vi "Intake Loop.vi"   [LabVIEW 2015]
uses:
  Common Code/Intake States.ctl
  Robot Global Data.vi
types:
  T1 = typedef "Dashboard Control Data.ctl" = cluster{"Shooter Presets":T2, "Encoder Control":T4, "Steer PID output":cluster{"output high":dbl, "output low":dbl}, " Steer PID gains":cluster{"proportional gain (Kc)":dbl, "integral time (Ti, min)":dbl, "derivative time (Td, min)":dbl}, "Drivetrain Settings":T5, "Vision Packet":T6, "Dashboard Drivetrain Command":T7, "Info/Command Cluster":T9, "Ball Vision Packet":T10, "Intake Presets":T12, "Intake Encoder Control":T14, "Climb Presets":T15, "Goal Output Range":cluster{"output high":dbl, "output low":dbl}, "Enabled Systems":T16, "Auton Presets":T17, "Pressure M":dbl, "Pressure B":dbl, "Vision Timeout":dbl}
  T2 = typedef "Shooter Presets.ctl" = cluster{"Batter Shot":T3, "Deep Middle":T3, "Manual Shot":T3, "Left Ticks Per Rotation":dbl, "Right Ticks Per Rotation":dbl, "Low Bar Shot":T3, "Shooter RPM Tolerance":dbl, "Trigger Power":dbl, "Fire from Load Delay":i32, "Max Angle":dbl, "Min Angle":dbl, "Angle PID gains":cluster{"P":dbl, "I":dbl, "D":dbl}, "Angle Output":cluster{"output high":dbl, "output low":dbl}, "Shooter Angle Tolerance":dbl, "Vision Shoot x^2":dbl, "Vision Shoot x":dbl, "Feed Forward Max Accel":dbl, "Feed Forward Kv":dbl, "Backwards Trigger":dbl, "Shot Finish Delay (ms)":dbl, "Angle Max Current":dbl, "Angle Current Trip Time":dbl, "Intake Angle":dbl, "Vision Shoot c":dbl, "Reset?":bool, "Button Release Delay":dbl, "Angle Pot x":dbl, "Angle Pot c":dbl, "Ignore Angle?":bool, "Max RPM":dbl, "Safty Frist Angle":dbl, "Intake Danger Height":dbl, "Angle Pot B":i32, "Angle Pot M":dbl, "FF Finish RPM":dbl, "RPM PID Right":cluster{"P":dbl, "I":dbl, "D":dbl, "FF":dbl}, "RPM PID Left":cluster{"P":dbl, "I":dbl, "D":dbl, "FF":dbl}, "Backwards RPM":dbl, "Vision RPM":dbl, "Run Wheels Backward Delay":u32, "Cleat Shot":T3}
  T3 = typedef "Shot Presets.ctl" = cluster{"L":dbl, "R":dbl, "A":dbl}
  T4 = typedef "Encoder Control.ctl" = cluster{"Right Tick Constant":dbl, "Left Tick Constant":dbl, "Reset?":bool, "Y Dist":cluster{"PID gains":cluster{"proportional gain (Kc)":dbl, "integral time (Ti, min)":dbl, "derivative time (Td, min)":dbl}}, "Y Stop Thresh":dbl, "Y Stop Speed":dbl}
  T5 = typedef "Drivetrain Settings.ctl" = cluster{"Gyro Tolerance":dbl, "Throttle Ramp (ms)":dbl, "Kv":dbl, "Ka":dbl, "Feed Forward P":dbl, "Feed Forward D":dbl, "Goal Vision PID gains":cluster{"proportional gain (Kc)":dbl, "integral time (Ti, min)":dbl, "derivative time (Td, min)":dbl}, "Goal Detection Window":dbl, "Creep Rate":dbl, "Vision Throttle Threshold":dbl, "Min Turn Output":dbl, "Left Batter Angle":dbl, "Right Batter Angle":dbl}
  T6 = typedef "Goal Vision Packet.ctl" = cluster{"Distance":dbl, "Center X":dbl, "Center Y":dbl, "Found Target?":bool, "Robot Center":dbl, "Angle":dbl}
  T7 = typedef "Dashboard Drivetrain Command.ctl" = cluster{"Drivetrain Vision":T8}
  T8 = typedef "Drivetrain Vision.ctl" = cluster{"Goal Window":dbl, "Ball Window":dbl}
  T9 = typedef "Ball Tracking Command Cluster.ctl" = cluster{"Distance to Ball":dbl, "Desired Angle":dbl, "Command":enum16{"Turn to Ball", "Turn to Angle", "Get Distance"}, "Pixels from Center":dbl}
  T10 = typedef "Ball Vision Packet.ctl" = cluster{"Ball Detected?":bool, "Distance to Ball":dbl, "Desired Angle":dbl, "Pixels from Center":dbl, "Tracking mode":T11}
  T11 = typedef "Tracking Mode.ctl" = enum16{"Turn to Ball", "Turn to Angle"}
  T12 = typedef "Intake Presets.ctl" = cluster{"Intake Speed":dbl, "Outake Speed":dbl, "Low Height":dbl, "Half Height":dbl, "Full Height":dbl, "Angle Speed":dbl, "Angle Tolerance":dbl, "Encoder Scale":dbl, "Load Height":dbl, "Output Range":T13, "Rotation Power Max/Min":dbl, "MaxCurrent":dbl, "Intake Trip Time":dbl, "Idle Height":dbl, "Max Height":dbl, "Reset Encoders?":bool, "PID gains":cluster{"proportional gain (Kc)":dbl, "integral time (Ti, min)":dbl, "derivative time (Td, min)":dbl}, "Intake Stop Delay":u32, "Settle Time":dbl, "Settle Wait Time":dbl}
  T13 = typedef "Drivetrain Output Range.ctl" = cluster{"output high":dbl, "output low":dbl}
  T14 = typedef "IntakeEcoderControl.ctl" = cluster{"Arm Tick Constant":dbl, "Reset?":bool, "Y Dist":cluster{"PID gains":cluster{"proportional gain (Kc)":dbl, "integral time (Ti, min)":dbl, "derivative time (Td, min)":dbl}}, "Y Stop Thresh":dbl, "Y Stop Speed":dbl}
  T15 = typedef "Climb Presets.ctl" = cluster{"Pull Power":dbl, "Extend Power":dbl}
  T16 = typedef "Enabled Systems.ctl" = cluster{"Shoot":bool, "Intake":bool, "DT":bool, "Gyro":bool, "100ms":bool, "US":bool}
  T17 = typedef "Autonomous Presets.ctl" = cluster{"Pitch Limit":dbl, "Roll Limit":dbl, "Start Position":dbl, "Cross Position":dbl}
  T18 = typedef "Intake Commands Cluster.ctl" = cluster{"Intake Commands":T19, "Intake Mode":T20, "Override IR":bool, "Angle Target":dbl}
  T19 = typedef "Intake Commands.ctl" = enum16{"Settle Ball", "Unload", "Load", "Pull up", "Drop low", "Idle", "Lift Half", "Go To Angle"}
  T20 = typedef "Intake Mode.ctl" = enum16{"Safe", "Auto", "Manual"}
  T21 = typedef "WPI_MotorControlDeviceRef.ctl" = cluster{"DeviceStatus":errorcluster, "Type":T22, "PWM":cluster{"PWM Channel":T23, "DeadBand":T24}, "CAN":cluster{"Device Number":u8, "Control Mode":T25, "Semaphore":T26, "Max Vout":dbl, "TalonSRX Control Mode":T27}, "Invert":bool}
  T22 = typedef "WPI_MotorControlType.ctl" = enum16{"PWM", "CAN", "CANTalonSRX"}
  T23 = typedef "FPGA_DIOPWMChannel.ctl" = enum8{"PWM 0", "PWM 1", "PWM 2", "PWM 3", "PWM 4", "PWM 5", "PWM 6", "PWM 7", "PWM 8", "PWM 9", "PWM MXP 0", "PWM MXP 1", "PWM MXP 2", "PWM MXP 3", "PWM MXP 4", "PWM MXP 5", "PWM MXP 6", "PWM MXP 7", "PWM MXP 8", "PWM MXP 9", "Invalid"}
  T24 = typedef "WPI_PWMDeadband.ctl" = cluster{"Name":string, "maxPositivePwm":i32, "minPositivePwm":i32, "centerPwm":i32, "maxNegativePwm":i32, "minNegativePwm":i32, "angularRange":u16}
  T25 = typedef "WPI_CANJaguar_ControlMode.ctl" = enum8{"Percent VBus", "Current", "Speed", "Position", "Voltage"}
  T26 = typedef "Semaphore RefNum" = refnum<k1>
  T27 = typedef "WPI_CANTalonSRX_APIControlMode.ctl" = enum8{"Percent VBus", "Speed", "Position", "Slave", "Unchanged / Invalid", "Voltage Compensation", "Current", "Motion Profile"}
  T28 = typedef "WPI_CANTalonSRX_GlobalStatus.ctl" = cluster{"Applied Throttle":dbl, "Module Enabled":bool, "CAN Error":errorcluster, "Closed Loop Error":dbl, "Forward Limit Switch Closed":bool, "Reverse Limit Switch Closed":bool, "Sensor Position":dbl, "Sensor Velocity":dbl, "Current":dbl, "Sticky Fault - Over Temp":bool, "Sticky Fault - Under Voltage":bool, "Sticky Fault - Forward Limit":bool, "Sticky Fault - Reverse Limit":bool, "Sticky Fault - Forward Soft Limit":bool, "Sticky Fault - Reverse Soft Limit":bool, "Brake is Enabled":bool, "Encoder Position":dbl, "Encoder Velocity":dbl, "Encoder Index Count":dbl, "Encoder A Pin State":bool, "Encoder B Pin State":bool, "Encoder Index Pin State":bool, "Analog In":dbl, "Analog In Velocity":dbl, "Temperature (C)":dbl, "Battery Voltage":dbl, "Control 5 Is Supported":bool, "Current Profile Slot Select":dbl, "Pos Div 8":bool, "Vel Div 4":bool, "Pulse Width Position":i32, "Pulse Width Velocity":i32, "Pulse Width Rise To Rise (us)":i32, "Pulse Width Rise To Fall (us)":i32, "Mot Prof Active Is Under Run":bool, "Mot Prof Active Has Under Run":bool, "Mot Prof Active Is Last":bool, "Mot Prof Active Velocity Only":bool, "Mot Prof Active Is Valid":bool, "Mot Prof Buffer Is Full":bool, "Mot Prof Active Profile Slot Select":i32, "Mot Prof NextID":i32, "Mot Prof Count":i32, "Mot Prof Active Velocity":dbl, "Mot Prof Active Position":dbl, "Mot Prof Output Enable":i32}
  T29 = typedef "Intake States.ctl" = enum16{"Idle", "Set roller speed", "Move to angle", "Go Hard or Go Home", "Ball Settle"}
  T30 = typedef "Intake Status Cluster.ctl" = cluster{"Roller Power":dbl, "Angle Power":dbl, "Intake Mode":T20, "Intake States":T29, "Rollers Active?":bool, "Current Height":dbl, "Target Height":dbl, "Encoder Raw Position":dbl, "Forward Tripped?":bool, "Backward Tripped?":bool, "Override IR?":bool}
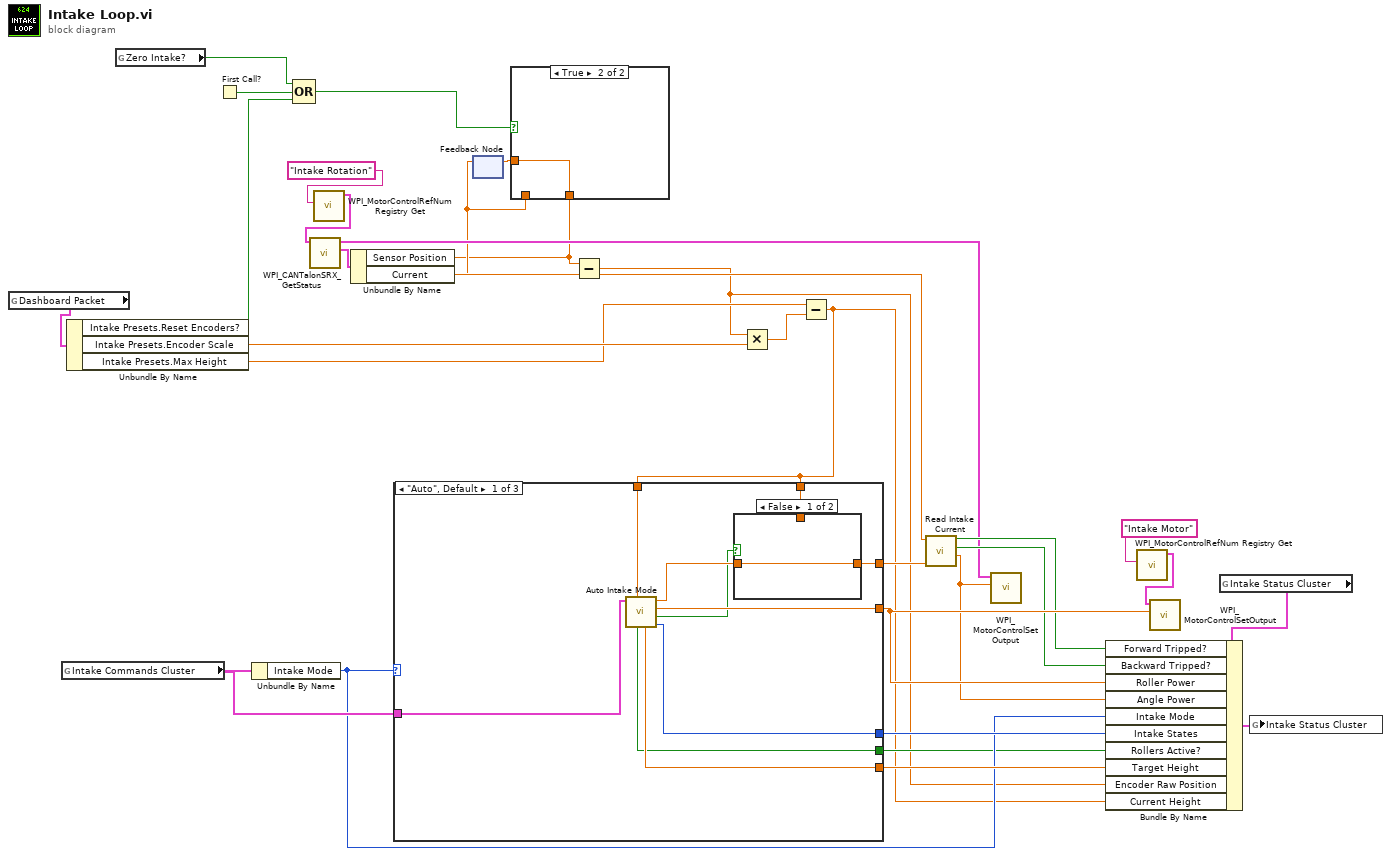
[diagram p0: block diagram]
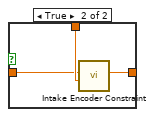
[diagram p3: hidden frame]
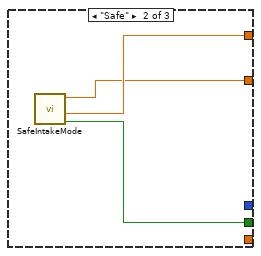
[diagram p4: hidden frame]
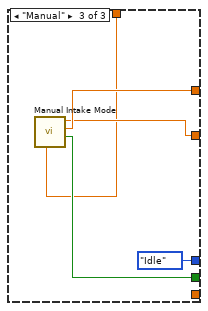
[diagram p5: hidden frame]
diagram:
  n1 = global read "Robot Global Data.vi" "Dashboard Packet"() -> (w14:T1)
  n2 = global read "Robot Global Data.vi" "Intake Commands Cluster"() -> (w32:T18)
  n3 = Unbundle By Name(w14) -> ("Intake Presets.Reset Encoders?"=w4:bool, "Intake Presets.Encoder Scale"=w16:dbl, "Intake Presets.Max Height"=w15:dbl)
  n4 = global read "Robot Global Data.vi" "Zero Intake?"() -> (w1:bool)
  n5 = First Call?() -> (First Call?: T/F=w3:bool)
  n6 = Unbundle By Name(w32) -> ("Intake Mode"=w25:T20)
  n7 = Compound Arithmetic op=OR(w1, w3, w4) -> (w2:bool)
  n8 = call <vilib>:"WPI_MotorControlRefNum Registry Get.vi"("refnum name"="Intake Rotation") -> ("MotorControlDevRef"=w10:T21)  [unwired: 9 in, 1 out]
  n9 = call <vilib>:"WPI_CANTalonSRX_GetStatus.vi"("CAN Talon SRX Ref"=w10) -> ("Talon SRX Status"=w13:T28, "CAN Talon SRX Ref"=w12:T21)  [unwired: 8 in, 1 out]
  n10 = Unbundle By Name(w13) -> ("Sensor Position"=w7:dbl, "Current"=w11:dbl)
  n11 = feedback #1() -> (w8:dbl)  [unwired: 1 in]
  n12 = case shown="True" w2 {
    tunnel: w7 -> [_ w34]
    tunnel: [w33 w34] -> w9
    tunnel: w8 -> [w33 _]
    frame False {
    }
    frame True {
    }
  }
  n13 = feedback-in #1(w9) -> ()
  n14 = Subtract(x=w7, y=w8) -> (x-y=w6:dbl)
  n15 = Multiply(x=w6, y=w16) -> (x*y=w17:dbl)
  n16 = Subtract(x=w15, y=w17) -> (x-y=w5:dbl)
  n17 = case shown="\"Auto\", Default" w25 {
    tunnel: w32 -> [w44 _ _]
    tunnel: [w37 w51 w55] -> w22
    tunnel: [w38 w50 w54] -> w29
    tunnel: [w42 _ Intake_States."Idle" ("Intake States")] -> w27
    tunnel: [w43 _ _] -> w26
    tunnel: w5 -> [w41 _ w52]
    tunnel: [w40 w49 w53] -> w18
    tunnel: w5 -> [w36 _ _]
    frame "Auto", Default {
      n18 = call "Auto Intake Mode.vi"("Intake Angle"=w36, "Intake Commands Cluster"=w44) -> ("Intake States"=w42:T29, "Limit with Encoders?"=w35:bool, "Roller Power"=w38:dbl, "Angle Power"=w39:dbl, "Target Height"=w43:dbl, "Rollers Active?"=w40:bool)  [unwired: 3 in, 1 out]
      n19 = case shown="False" w35 {
        tunnel: w41 -> [_ w48]
        tunnel: w39 -> [w45 w47]
        tunnel: [w45 w46] -> w37
        frame False {
        }
        frame True {
          n20 = call "Intake Encoder Constraint.vi"("Arm Power"=w47, "Encoder Position"=w48) -> ("Roller Power"=w46:dbl)  [unwired: 8 in]
        }
      }
    }
    frame "Safe" {
      n21 = call "SafeIntakeMode.vi"() -> ("Rollers Active?"=w49:bool, "Angle Power"=w51:dbl, "Roller Power"=w50:dbl)  [unwired: 9 in]
    }
    frame "Manual" {
      n22 = call "Manual Intake Mode.vi"("Current Encoder Position"=w52) -> ("Rollers Active?"=w53:bool, "Arm Power"=w55:dbl, "Intake Power"=w54:dbl)  [unwired: 8 in]
    }
  }
  n23 = call "Read Intake Current.vi"("Proposed Power"=w22, "Current"=w11) -> ("Actual Power"=w21:dbl, "Reverse Trip?"=w19:bool, "Forward Trip?"=w20:bool)  [unwired: 7 in]
  n24 = call <vilib>:"WPI_MotorControlSetOutput.vi"("Output"=w21, "MotorControlDevRef"=w12) -> ()  [unwired: 7 in, 3 out]
  n25 = call <vilib>:"WPI_MotorControlRefNum Registry Get.vi"("refnum name"="Intake Motor") -> ("MotorControlDevRef"=w30:T21)  [unwired: 9 in, 1 out]
  n26 = call <vilib>:"WPI_MotorControlSetOutput.vi"("Output"=w29, "MotorControlDevRef"=w30) -> ()  [unwired: 7 in, 3 out]
  n27 = global read "Robot Global Data.vi" "Intake Status Cluster"() -> (w24:T30)
  n28 = Bundle By Name(cluster=w24, "Forward Tripped?"=w20, "Backward Tripped?"=w19, "Roller Power"=w29, "Angle Power"=w21, "Intake Mode"=w25, "Intake States"=w27, "Rollers Active?"=w18, "Target Height"=w26, "Encoder Raw Position"=w6, "Current Height"=w5) -> (w28:T30)
  n29 = global write "Robot Global Data.vi" "Intake Status Cluster"(w28) -> ()
